vi "Util_RPMtoMPS.vi"(10 "rpm gear":dbl) -> (2 "m/s robot":dbl)   [LabVIEW 2009, in "OWNCAN.lvlib"]
uses:
  OWNCAN.lvlib
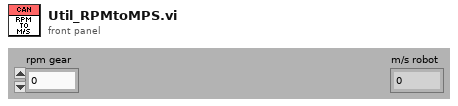
[diagram p1: front panel]
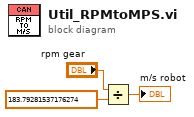
[diagram p0: block diagram]
diagram:
  n1 = Divide(x="rpm gear", y=183.79281537176274) -> (x/y=→"m/s robot":dbl)
